vi "Obtain Lock.vi"(8 "error in (no error)":errorcluster, 9 "timeout (-1 ms)":i32=-1 format="%d ms", 11 "Pointer in":refnum<class "Pointer.lvclass">) -> (0 "error out":errorcluster, 1 "timed out?":bool, 2 "lock status":bool, 3 "Pointer out":refnum<class "Pointer.lvclass">)   [LabVIEW 2017, in "Memory Manager.lvlib" / "Pointer.lvclass"]
uses:
  Pointer.lvclass
  Pointer.lvclass/Pointer.ctl
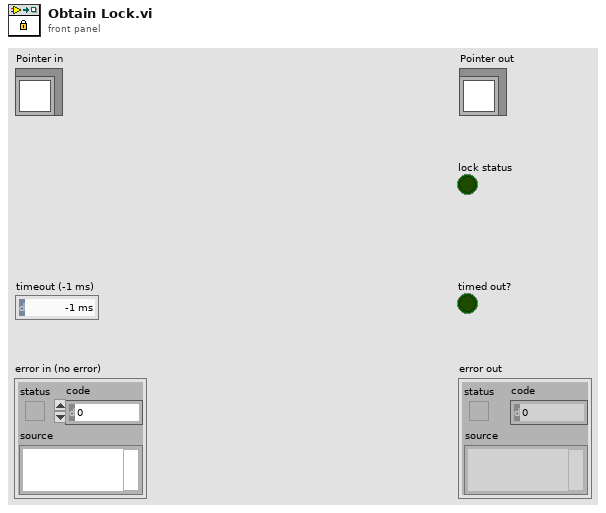
[diagram p1: front panel]
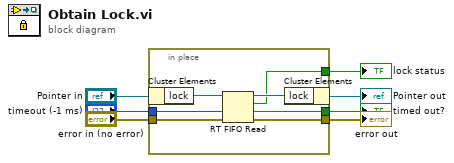
[diagram p0: block diagram]
diagram:
  n1 = in-place {
    in-place-border: "error in (no error)" -> [w14]
    in-place-border: [w13] -> w5
    in-place-border: "timeout (-1 ms)" -> [w12]
    in-place-border: [w11] -> w3
    in-place-border: [w8] -> w2
    n2 = in-place-cluster #1("Pointer in") -> ("lock"=w10:refnum<k33>)
    n3 = RT FIFO Read(0:w10, 2:w12, 3:w14) -> (8:w9:refnum<k33>, 9:w8:bool, 10:w11:bool, 11:w13:errorcluster)  [unwired: 1 in, 1 out]
    n4 = in-place-cluster #1("lock"=w9) -> (→"Pointer out":refnum<class "Pointer.lvclass">)
  }
  "error out" <- w5
  "timed out?" <- w3
  "lock status" <- w2
